vi "Update Pin Information.vi"(8 "error in":errorcluster, 9 "channel":string, 10 "pin_name":string, 11 "instrument object in":refnum<class "Abstract_Instrument.lvclass">) -> (0 "error out":errorcluster, 3 "instrument object out":refnum<class "Abstract_Instrument.lvclass">)   [LabVIEW 2021, in "Abstract_Instrument.lvclass"]
uses:
  Abstract_Instrument.lvclass
  Abstract_Instrument.lvclass/Abstract_Instrument.ctl
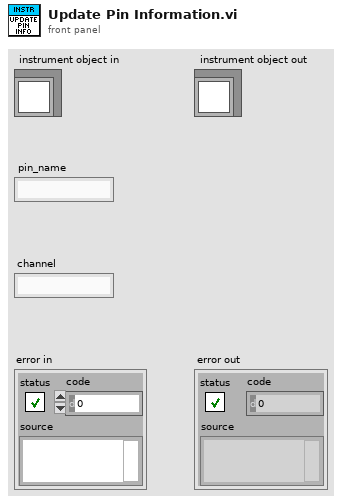
[diagram p1: front panel]
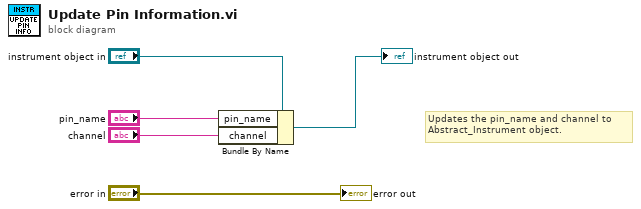
[diagram p0: block diagram]
diagram:
  # "Updates the pin_name and channel to \nAbstract_Instrument object."
  n1 = Bundle By Name(cluster="instrument object in", "pin_name"="pin_name", "channel"="channel") -> (→"instrument object out":refnum<class "Abstract_Instrument.lvclass">)
  "error out" <- "error in"
